vi "Check Stream Status.vi"(0 "niUsrpRio Session":T1={"Global Settings Register Bus"=refnum, "Radio 0 Settings Register Bus"=refnum, "Rx NI-USRP session"="", "Tx NI-USRP session"="", "FPGA Interface"=refnum, "RIO Interface Number"=0, "EEPROM Header"={"Checksum"=0, "Product Code"=0, "Hardware Current Version"=0, "Hardware Oldest Compatible Version"=0, "EEPROM Map Current Version"=0, "EEPROM Map Oldest Compatible Version"=0, "User Password"="", "Pointer to Factory Header"=0, "Pointer to User Header"=0, "Recommended Interval"=0, "Number of Reserved Bytes"=9, "Number of Daughterboards"=0, "Daughterboard IDs"=[], "Daughterboard Serial Numbers"=[]}, "Device Data Header"={"Checksum"=0, "Number of Channels"=0, "Number of Gain Settings"=[], "Pointer to Characterization Data"=[], "Number of Reserved Bytes"=27, "Number of Frequencies"=[]}, "EEPROM Characterization Header"={"Checksum"=0, "Date"=timestamp(0 s since 1904-01-01), "Temperature"=0.0, "Misc. Info"="", "Pointer to Device Data Header"=0, "Number of Reserved Bytes"=28}, "Characterization Data"=[], "Characterization Data Valid?"=FALSE, "Radio 1 Settings Register Bus"=refnum, "Radio Settings Bus Semaphore"=refnum} {"Characterization Data"."Frequencies [Hz]" format="%#_6p"; "EEPROM Characterization Header"."Pointer to Device Data Header" format="%x"; "EEPROM Characterization Header"."Checksum" format="%x"; "Device Data Header"."Pointer to Characterization Data" format="%x"; "Device Data Header"."Checksum" format="%x"; "EEPROM Header"."Pointer to User Header" format="%x"; "EEPROM Header"."Pointer to Factory Header" format="%x"; "EEPROM Header"."Product Code" format="%x"; "EEPROM Header"."Checksum" format="%x"}, 1 "scope":string(combo)="rx", 11 "error in":errorcluster, 12 "reference frequency source":string(combo)="Internal" caption="Reference Frequency Source") -> (4 "niUsrpRio Session (out)":T1={"Global Settings Register Bus"=refnum, "Radio 0 Settings Register Bus"=refnum, "Rx NI-USRP session"="", "Tx NI-USRP session"="", "FPGA Interface"=refnum, "RIO Interface Number"=0, "EEPROM Header"={"Checksum"=0, "Product Code"=0, "Hardware Current Version"=0, "Hardware Oldest Compatible Version"=0, "EEPROM Map Current Version"=0, "EEPROM Map Oldest Compatible Version"=0, "User Password"="", "Pointer to Factory Header"=0, "Pointer to User Header"=0, "Recommended Interval"=0, "Number of Reserved Bytes"=9, "Number of Daughterboards"=0, "Daughterboard IDs"=[], "Daughterboard Serial Numbers"=[]}, "Device Data Header"={"Checksum"=0, "Number of Channels"=0, "Number of Gain Settings"=[], "Pointer to Characterization Data"=[], "Number of Reserved Bytes"=27, "Number of Frequencies"=[]}, "EEPROM Characterization Header"={"Checksum"=0, "Date"=timestamp(0 s since 1904-01-01), "Temperature"=0.0, "Misc. Info"="", "Pointer to Device Data Header"=0, "Number of Reserved Bytes"=28}, "Characterization Data"=[], "Characterization Data Valid?"=FALSE, "Radio 1 Settings Register Bus"=refnum, "Radio Settings Bus Semaphore"=refnum} {"Characterization Data"."Frequencies [Hz]" format="%#_6p"; "EEPROM Characterization Header"."Pointer to Device Data Header" format="%x"; "EEPROM Characterization Header"."Checksum" format="%x"; "Device Data Header"."Pointer to Characterization Data" format="%x"; "Device Data Header"."Checksum" format="%x"; "EEPROM Header"."Pointer to User Header" format="%x"; "EEPROM Header"."Pointer to Factory Header" format="%x"; "EEPROM Header"."Product Code" format="%x"; "EEPROM Header"."Checksum" format="%x"}, 6 "done":bool caption="Done", 15 "error out":errorcluster)   [LabVIEW 2013]
doc: "Checks the status of the stream for when it is done, for FIFO overflows, for FIFO underflows, for DSP overflows, and if the clocks ever became unlocked. Checks the stream status after each Fetch Rx Data/Write Tx Data.\n\n<B>Input Parameters</B>\n\n<B>niUsrpRio Session</B> is the object created by the Open VI and used as the session handle for the USRP RIO design library.\n\n<B>Reference Frequency Source</B> is used when the source is GPS to determine whether to check if the GPS became unlocked.\n\n<B>scope</B> is the channel to check the stream status. The options are \"rx/RF 0\", \"rx/RF 1\", \"tx/RF 0\", and \"tx/RF 1\".\n\n<B>error in</B> describes error conditions that occur before this node runs. This input provides standard 'error in' functionality.\n\n<B>Output Parameters</B>\n\n<B>niUsrpRio Session (out)</B> is the niUsrpRio session used in all subsequent USRP RIO design library host VIs.\n\n<B>Done</B> indicates when the acquisition/generation has completed.\n\n<B>error out</B> contains error information. This output provides standard 'error out' functionality."
uses:
  <instrlib>/niUsrpRio/Config/v1/Host/Public/niUsrpRio Session.ctl
  <instrlib>/_niInstr/Register Bus/v0/Host/Public/Register Bus Session.ctl
  <instrlib>/_niInstr/Register Bus/v0/Host/Private/Session Data.ctl
  <instrlib>/niUsrpRio/Config/v1/Host/Public/EEPROM Header.ctl
  <instrlib>/niUsrpRio/Config/v1/Host/Public/EEPROM Device Data Header.ctl
  <instrlib>/niUsrpRio/Config/v1/Host/Public/EEPROM Characterization Header.ctl
  <instrlib>/niUsrpRio/Config/v1/Host/Public/Characterization Data.ctl
  <instrlib>/niUsrpRio/Config/v1/Host/Public/IQ Imbalance.ctl
  <instrlib>/niUsrpRio/Config/v1/Host/Public/What to Query for.ctl
  Program Files (x86)/National Instruments/LabVIEW 2013/ProjectTemplates/Source/NI-USRP/Simple NI-USRP Streaming/FPGA/SubVIs/Stream Control State.ctl
  Tx FPGA VI Reference.ctl
  Rx FPGA VI Reference.ctl
  <vilib>/rvi/interface/common/niFpgaWaitOnOcc.vi
  <vilib>/rvi/errors/niLvFpgaAdjustHostInterfaceError.vi
  <vilib>/rvi/interface/nirviReadWriteControl/nirviReadWriteControl.xnode
  NiFpgaLv.dll
  <vilib>/rvi/interface/Simulation/niFpgaSimulationCallBeginRW.vi
  <instrlib>/niUsrpRio/Config/v1/Host/niUsrpRio Config v1 Host.lvlib
  <instrlib>/_niInstr/Register Bus/v0/Host/niInstr Register Bus v0 Host.lvlib
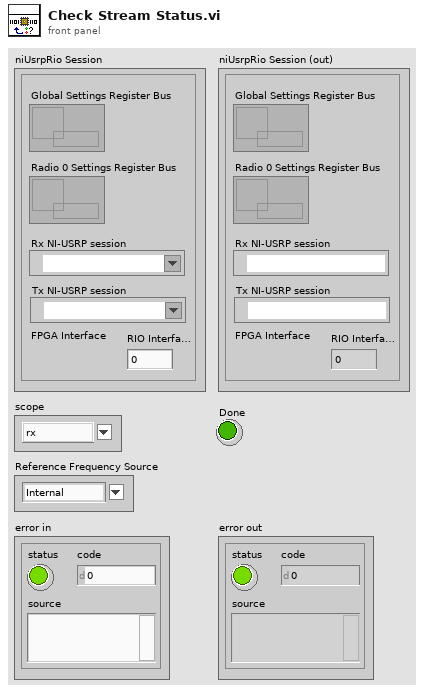
[diagram p1: front panel]
types:
  T1 = typedef "niUsrpRio Config v1 Host.lvlib/niUsrpRio Session.ctl" = cluster{"Global Settings Register Bus":T2, "Radio 0 Settings Register Bus":T2, "Rx NI-USRP session":refnum<k15>, "Tx NI-USRP session":refnum<k15>, "FPGA Interface":refnum<k20>, "RIO Interface Number":u32, "EEPROM Header":T3, "Device Data Header":T4, "EEPROM Characterization Header":T5, "Characterization Data":T6[], "Characterization Data Valid?":bool, "Radio 1 Settings Register Bus":T2, "Radio Settings Bus Semaphore":T8}
  T2 = typedef "niInstr Register Bus v0 Host.lvlib/Register Bus Session.ctl" = refnum<queue>
  T3 = typedef "niUsrpRio Config v1 Host.lvlib/EEPROM Header.ctl" = cluster{"Checksum":u32, "Product Code":u16, "Hardware Current Version":u16, "Hardware Oldest Compatible Version":u16, "EEPROM Map Current Version":u16, "EEPROM Map Oldest Compatible Version":u16, "User Password":string, "Pointer to Factory Header":u32, "Pointer to User Header":u32, "Recommended Interval":u16, "Number of Reserved Bytes":i32, "Number of Daughterboards":u8, "Daughterboard IDs":u16[], "Daughterboard Serial Numbers":string[]}
  T4 = typedef "niUsrpRio Config v1 Host.lvlib/EEPROM Device Data Header.ctl" = cluster{"Checksum":u32, "Number of Channels":u8, "Number of Gain Settings":u16[], "Pointer to Characterization Data":u32[], "Number of Reserved Bytes":i32, "Number of Frequencies":u16[]}
  T5 = typedef "niUsrpRio Config v1 Host.lvlib/EEPROM Characterization Header.ctl" = cluster{"Checksum":u32, "Date":timestamp, "Temperature":sgl, "Misc. Info":string, "Pointer to Device Data Header":u32, "Number of Reserved Bytes":i32}
  T6 = typedef "niUsrpRio Config v1 Host.lvlib/Characterization Data.ctl" = cluster{"Gains[dB]":dbl[], "Frequencies [Hz]":dbl[], "IQ Imbalance Table":T7[], "Measured Gains[dB]":dbl[][]}
  T7 = typedef "niUsrpRio Config v1 Host.lvlib/IQ Imbalance.ctl" = cluster{"Gain Imbalance [linear]":dbl, "Phase Imbalance [radians]":dbl, "Offset":cdb}
  T8 = typedef "Semaphore RefNum" = refnum<k1>
  T9 = typedef "niUsrpRio Config v1 Host.lvlib/What to Query for.ctl" = enum16{"Clock Chip Ever Unlocked", "LO Lock Status", "GPS Lock Status", "GPS Ever Unlocked"}
  T10 = typedef "Stream Control State.ctl" = enum16{"Idle", "Active"}
  T11 = typedef "niUsrpRio Config v1 Host.lvlib/Device Subfunction.ctl" = enum16{"rx", "tx"}
  T12 = typedef "niUsrpRio Config v1 Host.lvlib/RF Channel.ctl" = enum16{"0", "1", "All"}
  T13 = typedef "Tx FPGA VI Reference.ctl" = refnum<k20>
  T14 = typedef "Rx FPGA VI Reference.ctl" = refnum<k20>
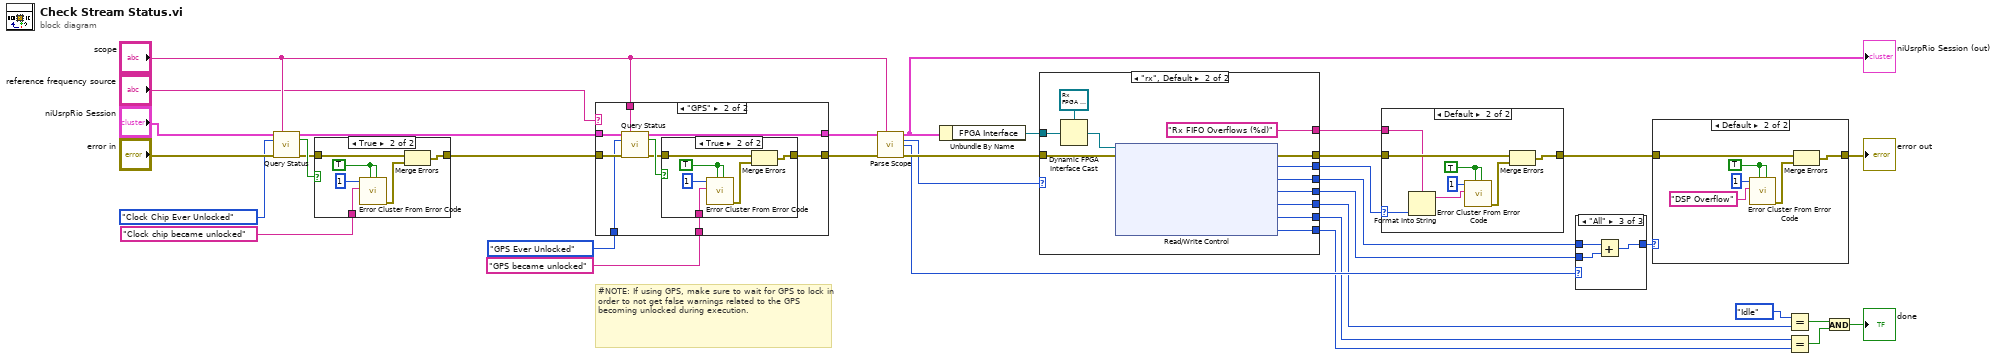
[diagram p0: block diagram]
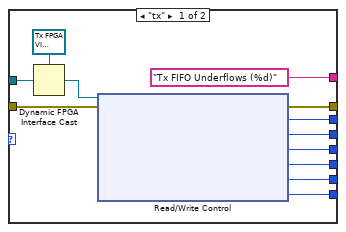
[diagram p9: hidden frame]
diagram:
  # "#NOTE: If using GPS, make sure to wait for GPS to lock in order to not get false warnings related to the GPS becoming unlocked during execution."
  n1 = call <instrlib>:"Query Status.vi"("niUsrpRio Session"="niUsrpRio Session", "scope"="scope", "What to Query for"=What_to_Query_for."Clock Chip Ever Unlocked", "Error In"="error in") -> ("niUsrpRio Session (out)"=w7:T1, "Status"=w29:bool, "Error Out"=w28:errorcluster)  [unwired: 9 in]
  n2 = case shown="True" w29 {
    tunnel: w28 -> [w35 w40]
    tunnel: [w35 w38] -> w9
    tunnel: "Clock chip became unlocked" ("error message (\"\")") -> [_ w36]
    frame False {
    }
    frame True {
      w37 = TRUE ("show call chain? (False)")
      n3 = call <vilib>:"Error Cluster From Error Code.vi"("is warning? (False)"=w37, "show call chain? (False)"=w37, "error message (\"\")"=w36, "error code (0)"=1) -> ("error out"=w39:errorcluster)  [unwired: 5 in]
      n4 = Merge Errors(w40, w39) -> (w38:errorcluster)
    }
  }
  n5 = case shown="\"GPS\"" "reference frequency source" {
    tunnel: w9 -> [w42 w52]
    tunnel: "scope" -> [_ w51]
    tunnel: w7 -> [w43 w50]
    tunnel: What_to_Query_for."GPS Ever Unlocked" ("What to Query for") -> [_ w49]
    tunnel: "GPS became unlocked" ("error message (\"\")") -> [_ w46]
    tunnel: [w43 w45] -> w1
    tunnel: [w42 w44] -> w2
    frame Default {
    }
    frame "GPS" {
      n6 = call <instrlib>:"Query Status.vi"("niUsrpRio Session"=w50, "scope"=w51, "What to Query for"=w49, "Error In"=w52) -> ("niUsrpRio Session (out)"=w45:T1, "Status"=w48:bool, "Error Out"=w47:errorcluster)  [unwired: 9 in]
      n7 = case shown="True" w48 {
        tunnel: w47 -> [w53 w58]
        tunnel: [w53 w56] -> w44
        tunnel: w46 -> [_ w54]
        frame False {
        }
        frame True {
          w55 = TRUE ("show call chain? (False)")
          n8 = call <vilib>:"Error Cluster From Error Code.vi"("is warning? (False)"=w55, "show call chain? (False)"=w55, "error message (\"\")"=w54, "error code (0)"=1) -> ("error out"=w57:errorcluster)  [unwired: 5 in]
          n9 = Merge Errors(w58, w57) -> (w56:errorcluster)
        }
      }
    }
  }
  n10 = call <instrlib>:"Parse Scope.vi"("niUsrpRio Session"=w1, "scope"="scope", "Error In"=w2) -> ("niUsrpRio Session (out)"=w24:T1, "Device Subfunction"=w23:T11, "Device Subfunction Channel"=w16:T12, "Error Out"=w34:errorcluster)  [unwired: 4 in, 5 out]
  "niUsrpRio Session (out)" <- w24
  n11 = Unbundle By Name(w24) -> ("FPGA Interface"=w32:refnum<k20>)
  n12 = case shown="\"rx\", Default" w23 {
    tunnel: w32 -> [w70 w83]
    tunnel: w34 -> [w69 w82]
    tunnel: [w67 w79] -> w21
    tunnel: [w66 w78] -> w22
    tunnel: [w65 w77] -> w18
    tunnel: [w64 w76] -> w17
    tunnel: [w63 w75] -> w14
    tunnel: [w62 w74] -> w13
    tunnel: [w61 w73] -> w12
    tunnel: ["Tx FIFO Underflows (%d)" ("error message (\"\")") "Rx FIFO Overflows (%d)" ("error message (\"\")")] -> w20
    frame "tx" {
      n13 = Dynamic FPGA Interface Cast(Session In=T13 refnum ("Type"), Type=w70) -> (Session Out=w68:T13)
      n14 = xnode "Read/Write Control"("FPGA VI Reference In"=w68, "error in"=w69) -> ("error out"=w66:errorcluster, "tx.underflows"=w67:u32, "tx 0.number of IQ data overflows"=w65:u64, "tx 1.number of IQ data overflows"=w64:u64, "tx.state"=w63:enum16{"Idle", "Active"}, "tx.samples processed"=w62:u32, "tx.samples to generate"=w61:u32)  [unwired: 1 out]
    }
    frame "rx", Default {
      n15 = Dynamic FPGA Interface Cast(Session In=T14 refnum ("Type"), Type=w83) -> (Session Out=w81:T14)
      n16 = xnode "Read/Write Control"("FPGA VI Reference In"=w81, "error in"=w82) -> ("error out"=w78:errorcluster, "rx.number of overflows"=w79:u32, "rx 0.number of IQ data overflows"=w77:u64, "rx 1.number of IQ data overflows"=w76:u64, "rx.state"=w75:enum16{"Idle", "Active"}, "rx.samples processed"=w74:u32, "rx.samples to acquire"=w73:u32)  [unwired: 1 out]
    }
  }
  n17 = case shown="Default" w21 {
    selector: w21 -> [_ w86]
    tunnel: w22 -> [w84 w91]
    tunnel: [w84 w89] -> w19
    tunnel: w20 -> [_ w85]
    frame 0 {
    }
    frame Default {
      w87 = TRUE ("show call chain? (False)")
      n18 = Format Into String(format string=w85, w86) -> (resulting string=w88:string)  [unwired: 2 in, 1 out]
      n19 = call <vilib>:"Error Cluster From Error Code.vi"("is warning? (False)"=w87, "show call chain? (False)"=w87, "error message (\"\")"=w88, "error code (0)"=1) -> ("error out"=w90:errorcluster)  [unwired: 5 in]
      n20 = Merge Errors(w91, w90) -> (w89:errorcluster)
    }
  }
  n21 = case shown="\"All\"" w16 {
    tunnel: w18 -> [w93 _ w97]
    tunnel: w17 -> [_ w94 w96]
    tunnel: [w93 w94 w95] -> w15
    frame "0", Default {
    }
    frame "1" {
    }
    frame "All" {
      n22 = Add(x=w97, y=w96) -> (x+y=w95:u64)
    }
  }
  n23 = case shown="Default" w15 {
    tunnel: w19 -> [w98 w102]
    tunnel: [w98 w100] -> w10
    frame 0 {
    }
    frame Default {
      w99 = TRUE ("show call chain? (False)")
      n24 = call <vilib>:"Error Cluster From Error Code.vi"("is warning? (False)"=w99, "show call chain? (False)"=w99, "error message (\"\")"="DSP Overflow" ("error message (\"\")"), "error code (0)"=1) -> ("error out"=w101:errorcluster)  [unwired: 5 in]
      n25 = Merge Errors(w102, w101) -> (w100:errorcluster)
    }
  }
  "error out" <- w10
  n26 = Equal?(x=Stream_Control_State."Idle" ("state"), y=w14) -> (x = y?=w27:bool)
  n27 = Equal?(x=w13, y=w12) -> (x = y?=w26:bool)
  n28 = And(x=w27, y=w26) -> (x .and. y?=→"done":bool)
